vi "VPA QC Get Data.vi"(8 "error in (no error)":errorcluster, 10 "DAQ Ref Cluster":T1) -> (0 "error out":errorcluster, 3 "IP Connected?":bool)   [LabVIEW 2013]
uses:
  Controls/VPA QC DAQ Ref Cluster.ctl
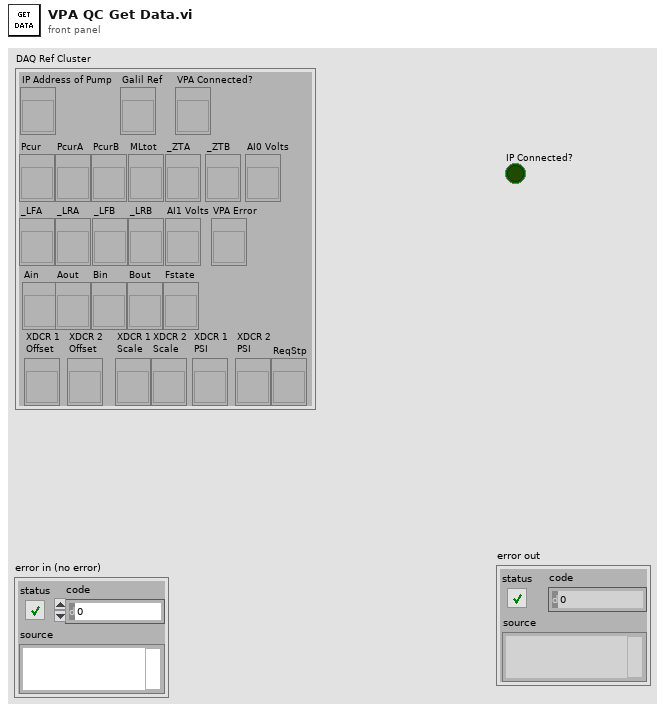
[diagram p1: front panel]
types:
  T1 = typedef "VPA QC DAQ Ref Cluster.ctl" = cluster{"IP Address of Pump":refnum<vi>, "Galil Ref":refnum<vi>, "VPA Connected?":refnum<vi>, "Pcur":refnum<vi>, "PcurA":refnum<vi>, "PcurB":refnum<vi>, "MLtot":refnum<vi>, "_LFA":refnum<vi>, "_LRA":refnum<vi>, "_LFB":refnum<vi>, "_LRB":refnum<vi>, "_ZTA":refnum<vi>, "_ZTB":refnum<vi>, "AI0 Volts":refnum<vi>, "AI1 Volts":refnum<vi>, "VPA Error":refnum<vi>, "Ain":refnum<vi>, "Aout":refnum<vi>, "Bin":refnum<vi>, "Bout":refnum<vi>, "Fstate":refnum<vi>, "XDCR 1\nOffset":refnum<vi>, "XDCR 2 \nOffset":refnum<vi>, "XDCR 1\nScale":refnum<vi>, "XDCR 2\nScale":refnum<vi>, "XDCR 1\nPSI":refnum<vi>, "XDCR 2\nPSI":refnum<vi>, "ReqStp":refnum<vi>}
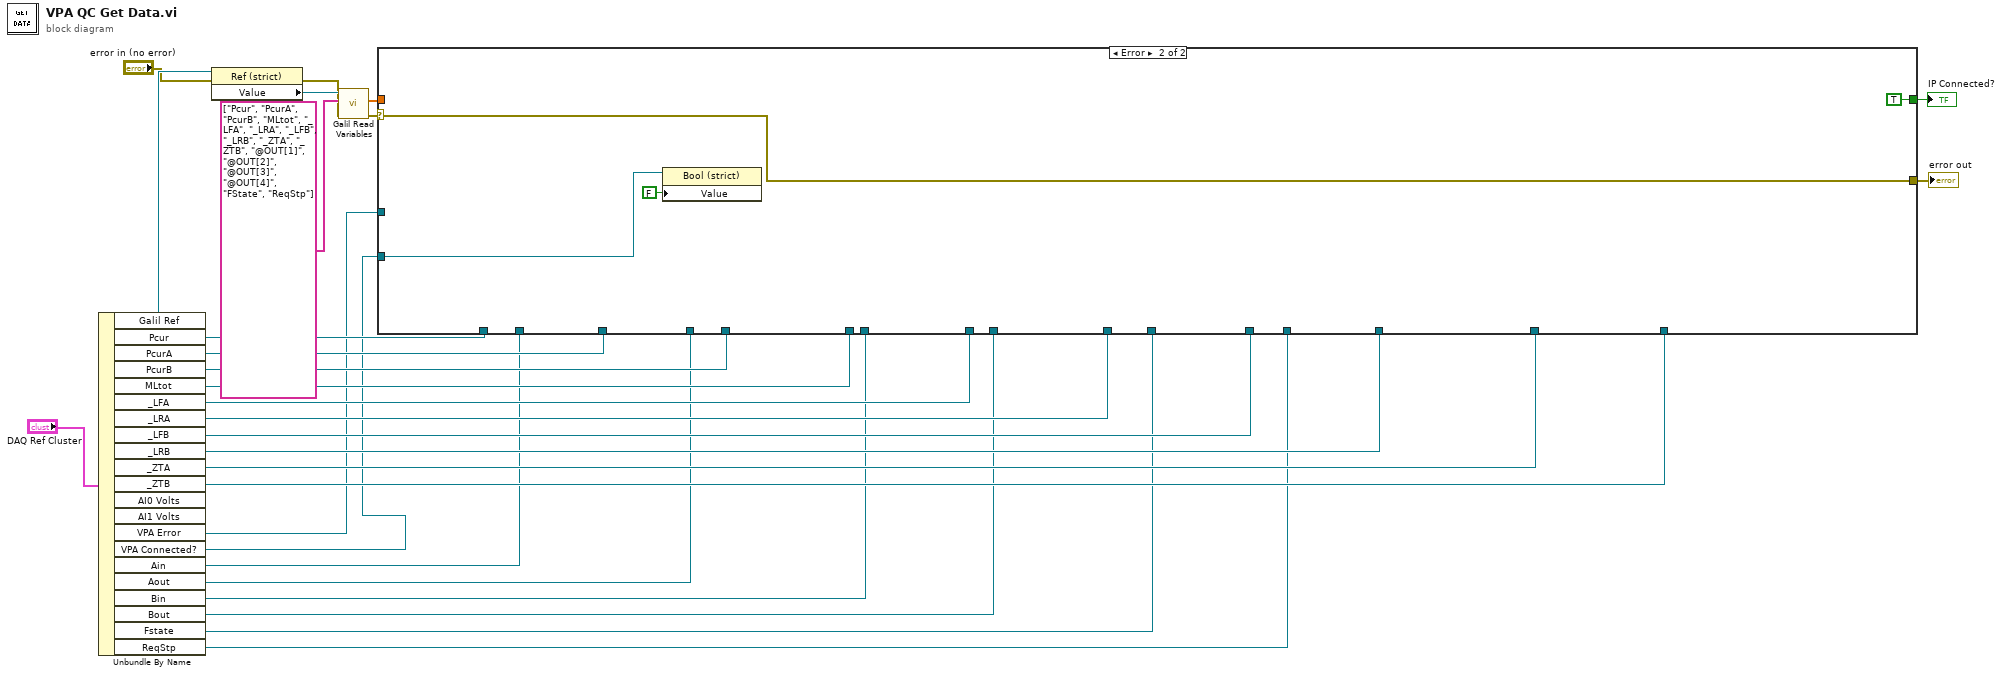
[diagram p0: block diagram]
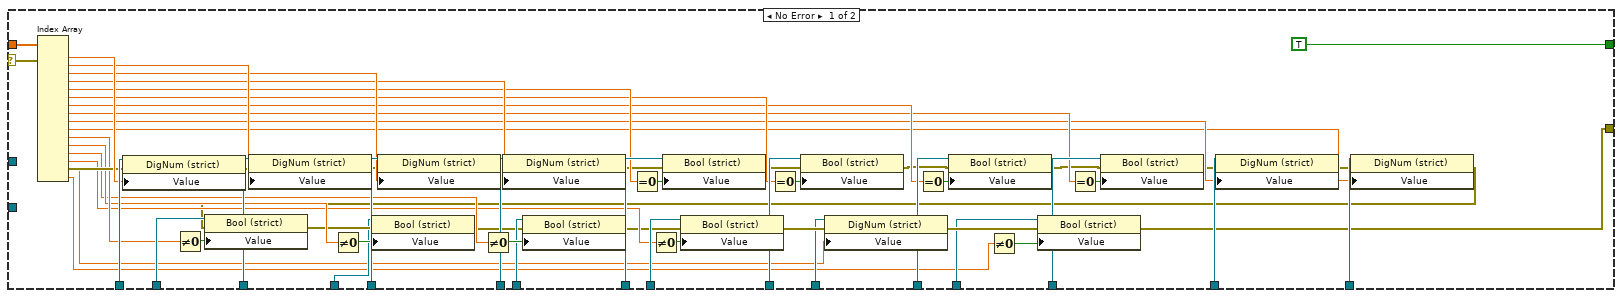
[diagram p2: hidden frame]
diagram:
  n1 = Unbundle By Name("DAQ Ref Cluster") -> ("Galil Ref"=w27:refnum<vi>, "Pcur"=w24:refnum<vi>, "PcurA"=w22:refnum<vi>, "PcurB"=w21:refnum<vi>, "MLtot"=w20:refnum<vi>, "_LFA"=w19:refnum<vi>, "_LRA"=w18:refnum<vi>, "_LFB"=w17:refnum<vi>, "_LRB"=w16:refnum<vi>, "_ZTA"=w15:refnum<vi>, "_ZTB"=w14:refnum<vi>, "VPA Error"=w11:refnum<vi>, "VPA Connected?"=w9:refnum<vi>, "Ain"=w7:refnum<vi>, "Aout"=w6:refnum<vi>, "Bin"=w5:refnum<vi>, "Bout"=w4:refnum<vi>, "Fstate"=w3:refnum<vi>, "ReqStp"=w1:refnum<vi>)  [unwired: 2 out]
  n2 = property class="Ref (strict)"(reference=w27, error in="error in (no error)") -> (error out=w13:errorcluster, "Value"=w26:refnum<k7>)  [unwired: 1 out]
  n3 = call "Galil Read Variables.vi"("error in (no error)"=w13, "Var Names"=string[] ["Pcur", "PcurA", "PcurB", "MLtot", "_LFA", "_LRA", "_LFB", "_LRB", "_ZTA", "_ZTB", "@OUT[1]", "@OUT[2]", "@OUT[3]", "@OUT[4]", "FState", "ReqStp"], "Automation Refnum in"=w26) -> ("error out"=w12:errorcluster, "Values"=w23:dbl[])  [unwired: 5 in, 2 out]
  n4 = case shown="Error" w12 {
    selector: w12 -> [w54 w89]
    tunnel: w24 -> [w88 _]
    tunnel: w23 -> [w87 _]
    tunnel: w22 -> [w85 _]
    tunnel: w21 -> [w83 _]
    tunnel: w20 -> [w81 _]
    tunnel: w19 -> [w79 _]
    tunnel: w18 -> [w75 _]
    tunnel: w17 -> [w72 _]
    tunnel: w16 -> [w69 _]
    tunnel: w15 -> [w67 _]
    tunnel: w14 -> [w65 _]
    tunnel: w11 -> [_ _]
    tunnel: [w31 w89] -> w2
    tunnel: w9 -> [_ w92]
    tunnel: [TRUE ("Value") TRUE ("Value")] -> w8
    tunnel: w7 -> [w52 _]
    tunnel: w6 -> [w37 _]
    tunnel: w5 -> [w46 _]
    tunnel: w4 -> [w45 _]
    tunnel: w3 -> [w35 _]
    tunnel: w1 -> [w32 _]
    frame No Error {
      n5 = Index Array(array=w87) -> (element #1=w86:dbl, element #2=w84:dbl, element #3=w82:dbl, element #4=w80:dbl, element #5=w77:dbl, element #6=w74:dbl, element #7=w71:dbl, element #8=w68:dbl, element #9=w66:dbl, element #10=w64:dbl, element #11=w47:dbl, element #12=w44:dbl, element #13=w43:dbl, element #14=w42:dbl, element #15=w34:dbl, element #16=w29:dbl)  [unwired: 16 in]
      n6 = property class="DigNum (strict)"(reference=w88, error in=w54, "Value"=w86) -> (error out=w63:errorcluster)  [unwired: 1 out]
      n7 = Not Equal To 0?(x=w47) -> (x != 0?=w51:bool)
      n8 = property class="DigNum (strict)"(reference=w85, error in=w63, "Value"=w84) -> (error out=w62:errorcluster)  [unwired: 1 out]
      n9 = Not Equal To 0?(x=w44) -> (x != 0?=w50:bool)
      n10 = property class="DigNum (strict)"(reference=w83, error in=w62, "Value"=w82) -> (error out=w61:errorcluster)  [unwired: 1 out]
      n11 = Not Equal To 0?(x=w43) -> (x != 0?=w49:bool)
      n12 = property class="DigNum (strict)"(reference=w81, error in=w61, "Value"=w80) -> (error out=w60:errorcluster)  [unwired: 1 out]
      n13 = Equal To 0?(x=w77) -> (x = 0?=w78:bool)
      n14 = Not Equal To 0?(x=w42) -> (x != 0?=w48:bool)
      n15 = property class="Bool (strict)"(reference=w79, error in=w60, "Value"=w78) -> (error out=w59:errorcluster)  [unwired: 1 out]
      n16 = Equal To 0?(x=w74) -> (x = 0?=w76:bool)
      n17 = property class="Bool (strict)"(reference=w75, error in=w59, "Value"=w76) -> (error out=w58:errorcluster)  [unwired: 1 out]
      n18 = Equal To 0?(x=w71) -> (x = 0?=w73:bool)
      n19 = property class="Bool (strict)"(reference=w72, error in=w58, "Value"=w73) -> (error out=w57:errorcluster)  [unwired: 1 out]
      n20 = Not Equal To 0?(x=w29) -> (x != 0?=w30:bool)
      n21 = Equal To 0?(x=w68) -> (x = 0?=w70:bool)
      n22 = property class="Bool (strict)"(reference=w69, error in=w57, "Value"=w70) -> (error out=w56:errorcluster)  [unwired: 1 out]
      n23 = property class="DigNum (strict)"(reference=w67, error in=w56, "Value"=w66) -> (error out=w55:errorcluster)  [unwired: 1 out]
      n24 = property class="DigNum (strict)"(reference=w65, error in=w55, "Value"=w64) -> (error out=w41:errorcluster)  [unwired: 1 out]
      n25 = property class="Bool (strict)"(reference=w52, error in=w41, "Value"=w51) -> (error out=w40:errorcluster)  [unwired: 1 out]
      n26 = property class="Bool (strict)"(reference=w37, error in=w40, "Value"=w50) -> (error out=w39:errorcluster)  [unwired: 1 out]
      n27 = property class="Bool (strict)"(reference=w46, error in=w39, "Value"=w49) -> (error out=w38:errorcluster)  [unwired: 1 out]
      n28 = property class="Bool (strict)"(reference=w45, error in=w38, "Value"=w48) -> (error out=w36:errorcluster)  [unwired: 1 out]
      n29 = property class="DigNum (strict)"(reference=w35, error in=w36, "Value"=w34) -> (error out=w33:errorcluster)  [unwired: 1 out]
      n30 = property class="Bool (strict)"(reference=w32, error in=w33, "Value"=w30) -> (error out=w31:errorcluster)  [unwired: 1 out]
    }
    frame Error {
      n31 = property class="Bool (strict)"(reference=w92, "Value"=FALSE) -> ()  [unwired: 1 in, 2 out]
    }
  }
  "error out" <- w2
  "IP Connected?" <- w8
